vi "delete subvi owner.vi"(8 "error in":errorcluster, 11 "Terminal in":refnum<vi>) -> (0 "error out":errorcluster, 3 "other terminals":refnum<vi>[](array[refnum]))   [LabVIEW 2013, in "TagBusProcessingPluginFeatureDecider.lvclass"]
uses:
  TagBusProcessingPluginFeatureDecider.lvclass
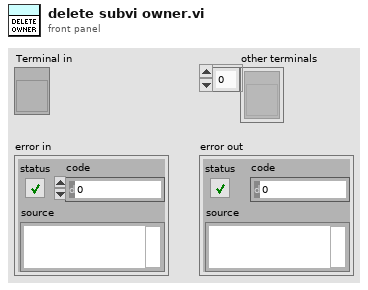
[diagram p1: front panel]
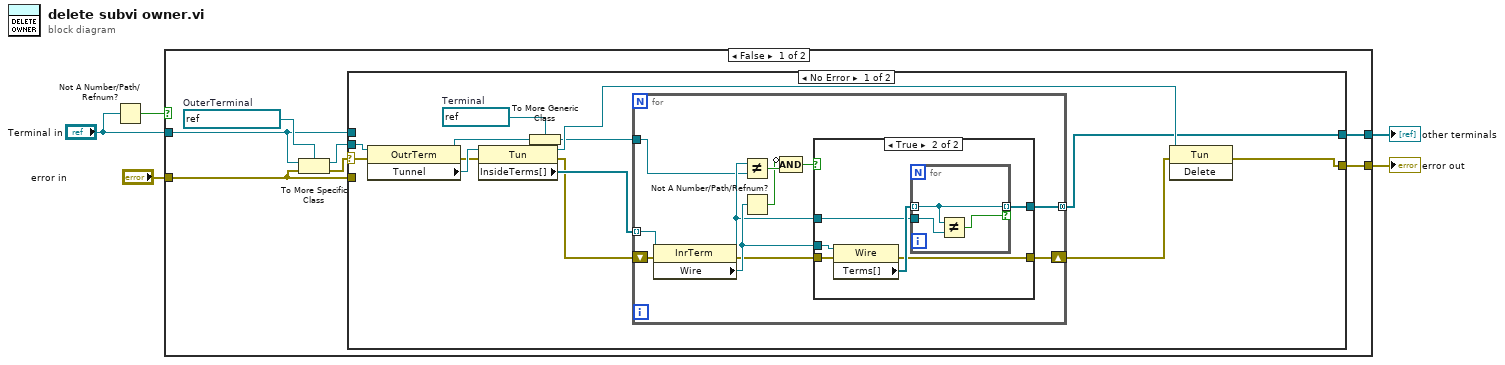
[diagram p0: block diagram]
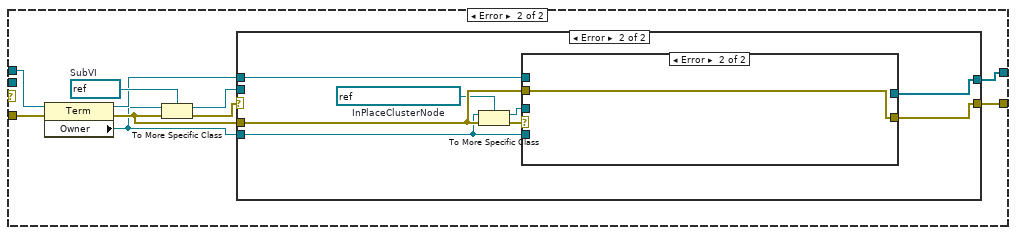
[diagram p3: hidden frame]
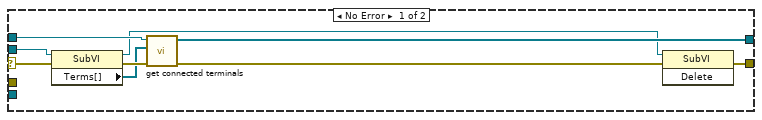
[diagram p4: hidden frame]
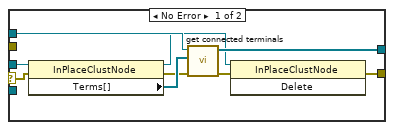
[diagram p5: hidden frame]
diagram:
  n1 = Not A Number/Path/Refnum?(number/path/refnum="Terminal in") -> (NaN/Path/Refnum?=w1:bool)
  n2 = case shown="False" w1 {
    tunnel: "error in" -> [w8 w84]
    tunnel: [w12 w84] -> w4
    tunnel: [w11 _] -> w3
    tunnel: "Terminal in" -> [w7 _]
    frame False {
      w10 = refnum<vi> refnum  # OuterTerminal
      n3 = To More Specific Class(target class=w10, reference=w7, error in=w8) -> (specific class reference=w6:refnum<vi>, error out=w9:errorcluster)
      n4 = case shown="No Error" w9 {
        selector: w9 -> [w24 _]
        tunnel: [w20 w53] -> w12
        tunnel: [w14 w50] -> w11
        tunnel: w8 -> [_ w48]
        tunnel: w7 -> [_ w47]
        tunnel: w6 -> [w25 _]
        frame No Error {
          w15 = refnum<vi> refnum  # Terminal
          n5 = property class="OutrTerm"(reference=w25, error in=w24) -> (reference out=w19:refnum<vi>, error out=w21:errorcluster, "Tunnel"=w22:refnum<vi>)
          n6 = property class="Tun"(reference=w22, error in=w21) -> (reference out=w23:refnum<vi>, error out=w17:errorcluster, "InsideTerms[]"=w18:refnum<vi>[])
          n7 = To More Generic Class(target class=w15, reference=w19) -> (generic class reference=w16:refnum<vi>)
          n8 = for {
            tunnel: w18 -> [w36] mode=indexing
            shift-right: [w30] -> w13
            shift-left: w17 -> [w35]
            tunnel: [w27] -> w14 mode=concatenating
            tunnel: w16 -> [w26]
            n9 = property class="InrTerm"(reference=w36, error in=w35) -> (reference out=w28:refnum<vi>, error out=w29:errorcluster, "Wire"=w31:refnum<vi>)
            n10 = Not Equal?(x=w28, y=w26) -> (x != y?=w34:bool)
            n11 = Not A Number/Path/Refnum?(number/path/refnum=w31) -> (NaN/Path/Refnum?=w33:bool)
            n12 = Compound Arithmetic op=AND(invert w33, w34) -> (w32:bool)
            n13 = case shown="True" w32 {
              tunnel: w31 -> [_ w43]
              tunnel: [w37 w38] -> w30
              tunnel: w29 -> [w37 w42]
              tunnel: w28 -> [_ w40]
              tunnel: [_ w39] -> w27
              frame False {
              }
              frame True {
                n14 = property class="Wire"(reference=w43, error in=w42) -> (error out=w38:errorcluster, "Terms[]"=w41:refnum<vi>[])  [unwired: 1 out]
                n15 = for {
                  tunnel: w41 -> [w45] mode=indexing
                  tunnel: w40 -> [w46]
                  tunnel: [w45] -> w39 mode=indexing if=w44
                  n16 = Not Equal?(x=w45, y=w46) -> (x != y?=w44:bool)
                }
              }
            }
          }
          n17 = invoke class="Tun" method="Delete"(reference=w23, error in=w13) -> (error out=w20:errorcluster)  [unwired: 1 in, 2 out]
        }
        frame Error {
          w54 = refnum<vi> refnum  # SubVI
          n18 = property class="Term"(reference=w47, error in=w48) -> (reference out=w51:refnum<vi>, error out=w56:errorcluster, "Owner"=w49:refnum<vi>)
          n19 = To More Specific Class(target class=w54, reference=w49, error in=w56) -> (specific class reference=w52:refnum<vi>, error out=w55:errorcluster)
          n20 = case shown="Error" w55 {
            selector: w55 -> [w57 _]
            tunnel: [w65 w70] -> w50
            tunnel: w51 -> [w62 w71]
            tunnel: w52 -> [w59 _]
            tunnel: [w58 w73] -> w53
            tunnel: w56 -> [_ w72]
            tunnel: w49 -> [_ w66]
            frame No Error {
              n21 = property class="SubVI"(reference=w59, error in=w57) -> (reference out=w60:refnum<vi>, error out=w63:errorcluster, "Terms[]"=w61:refnum<vi>[])
              n22 = call "get connected terminals.vi"("error in"=w63, "all terms"=w61, "excluded term"=w62) -> ("error out"=w64:errorcluster, "other terms"=w65:refnum<vi>[])  [unwired: 7 in]
              n23 = invoke class="SubVI" method="Delete"(reference=w60, error in=w64) -> (error out=w58:errorcluster)  [unwired: 1 in, 2 out]
            }
            frame Error {
              w69 = refnum<vi> refnum  # InPlaceClusterNode
              n24 = To More Specific Class(target class=w69, reference=w66, error in=w72) -> (specific class reference=w67:refnum<vi>, error out=w68:errorcluster)
              n25 = case shown="Error" w68 {
                selector: w68 -> [w80 _]
                tunnel: [w75 w83] -> w73
                tunnel: w72 -> [_ w83]
                tunnel: w71 -> [w82 _]
                tunnel: [w81 _] -> w70
                tunnel: w67 -> [w79 _]
                tunnel: w66 -> [_ _]
                frame No Error {
                  n26 = property class="InPlaceClustNode"(reference=w79, error in=w80) -> (reference out=w74:refnum<vi>, error out=w77:errorcluster, "Terms[]"=w78:refnum<vi>[])
                  n27 = call "get connected terminals.vi"("error in"=w77, "all terms"=w78, "excluded term"=w82) -> ("error out"=w76:errorcluster, "other terms"=w81:refnum<vi>[])  [unwired: 7 in]
                  n28 = invoke class="InPlaceClustNode" method="Delete"(reference=w74, error in=w76) -> (error out=w75:errorcluster)  [unwired: 1 in, 2 out]
                }
                frame Error {
                }
              }
            }
          }
        }
      }
    }
    frame True {
    }
  }
  "error out" <- w4
  "other terminals" <- w3
